vi "test_GetItemInformationFromProjects.vi"() -> (3 "Pass?":bool)   [LabVIEW 2019, in "Tests.SolutionBuilder.lvlib"]
uses:
  Tests.SolutionBuilder.lvlib
  SolutionBuilder/SolutionBuilder.lvclass
  SolutionBuilder/ProjectItem/ProjectItem.lvclass
panel:
  out "test results":u32 format="%03b"
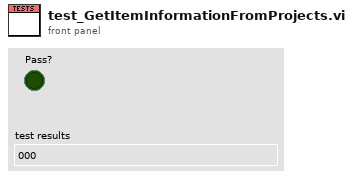
[diagram p1: front panel]
types:
  T1 = cluster{"Relative Path from 1 to 2":path, string[]}
  T2 = cluster{"Relative Path from 1 to 2":path, string[]}[]
  T3 = typedef "SolutionBuilder.lvlib/SolutionBuilder.lvclass/ProjectItemMap.ctl" = map{path, refnum<class "ProjectItem.lvclass">[]}
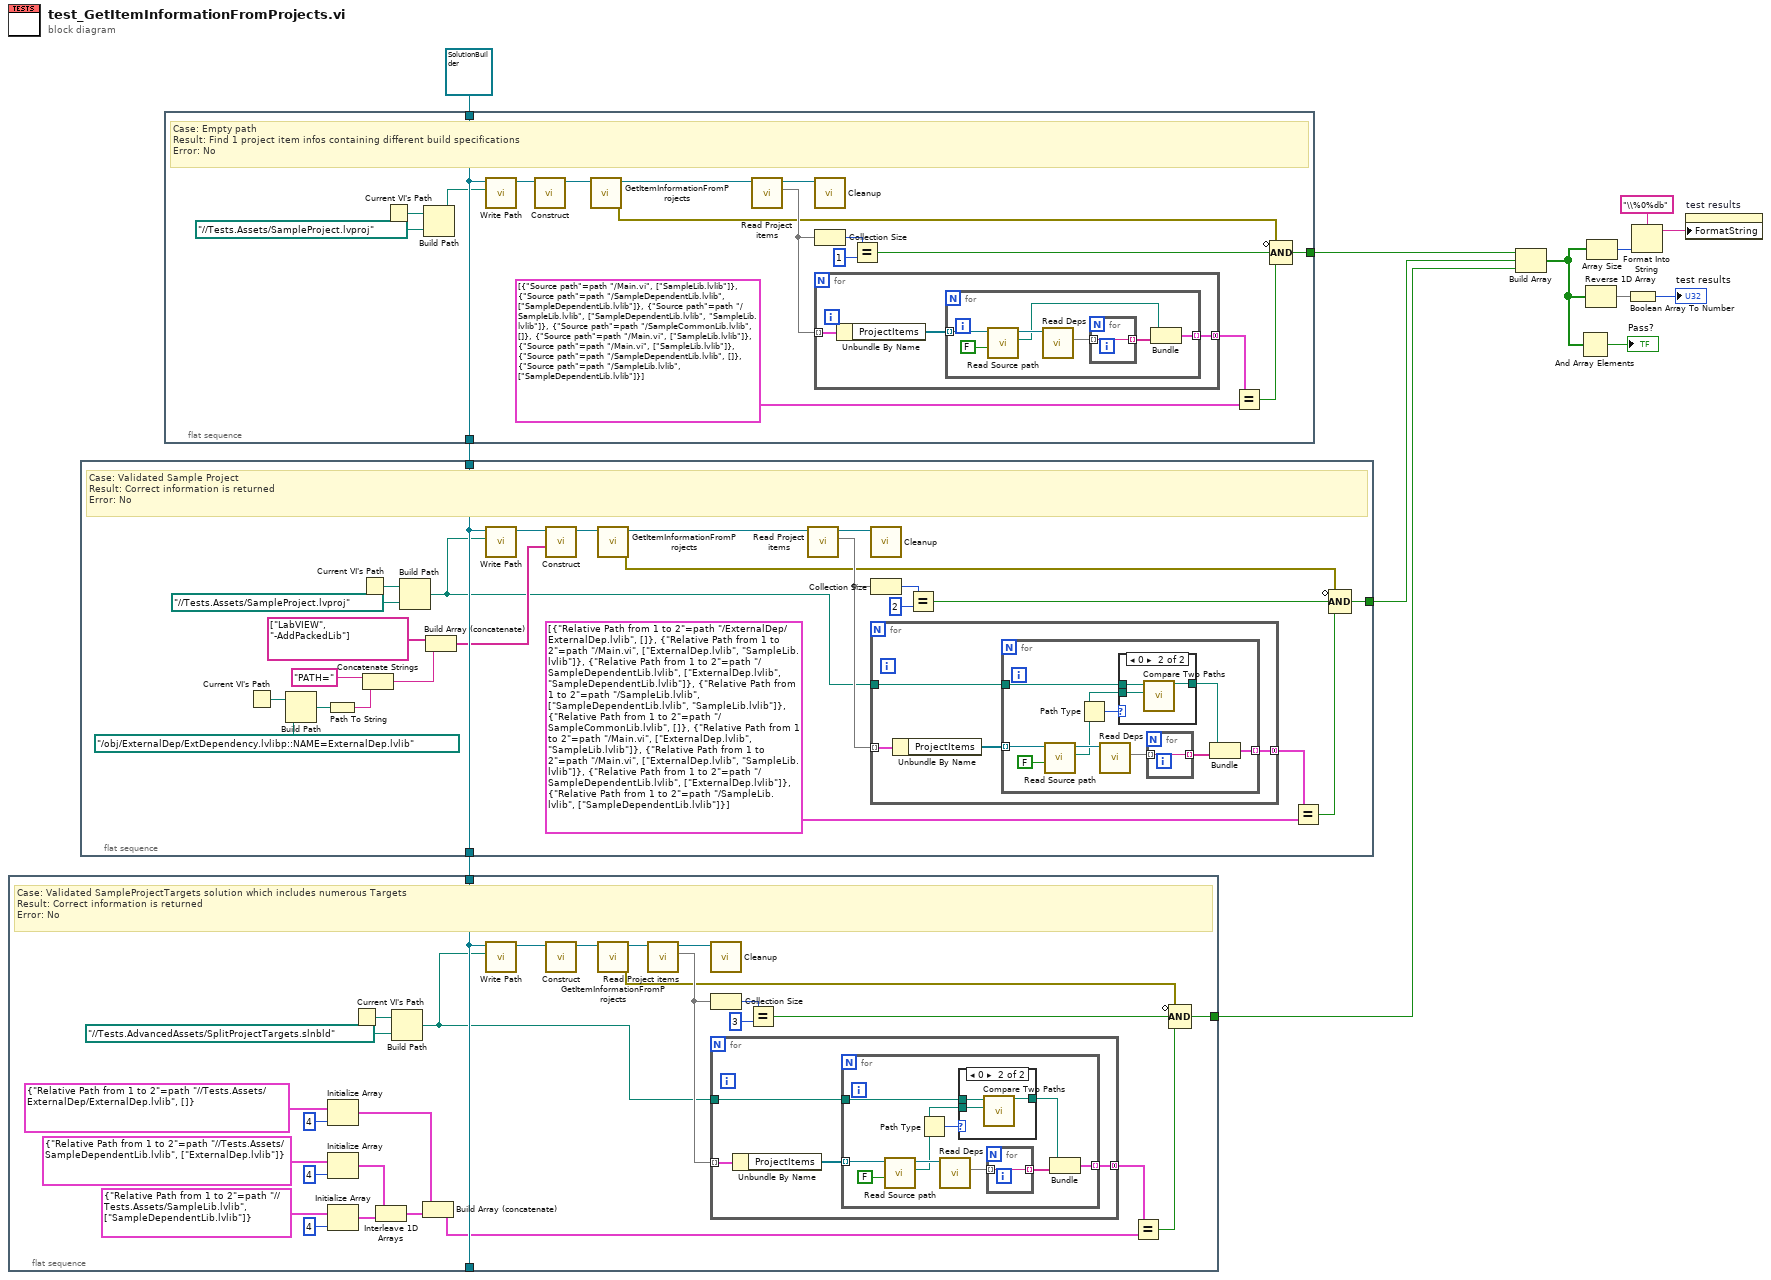
[diagram p0: block diagram]
diagram:
  n1 = flat-sequence {
    tunnel: [w33] -> w1
    tunnel: w2 -> [w40]
    tunnel: [w40] -> _
    frame #0 {
      # "Case: Validated SampleProjectTargets solution which includes numerous Targets\nResult: Correct information is returned\nError: No"
      n2 = Initialize Array(T1 {"Relative Path from 1 to 2"=path "../../Tests.Assets/ExternalDep/ExternalDep.lvlib", []}, 4 ("dimension size")) -> (w16:T2)
      n3 = Initialize Array(T1 {"Relative Path from 1 to 2"=path "../../Tests.Assets/SampleDependentLib.lvlib", ["ExternalDep.lvlib"]}, 4 ("dimension size")) -> (w18:T2)
      n4 = Initialize Array(T1 {"Relative Path from 1 to 2"=path "../../Tests.Assets/SampleLib.lvlib", ["SampleDependentLib.lvlib"]}, 4 ("dimension size")) -> (w17:T2)
      n5 = Current VI's Path() -> (path=w39:path)
      n6 = Interleave 1D Arrays(w18, w17) -> (w15:T2)
      n7 = Build Path(base path=w39, name or relative path=path "../../Tests.AdvancedAssets/SplitProjectTargets.slnbld" ("Path")) -> (appended path=w26:path)
      n8 = Build Array (concatenate)(w16, w15) -> (w14:T2)
      n9 = call-dynamic "Write Path.vi"("Path"=w26, "SolutionBuilder in"=w40) -> ("SolutionBuilder out"=w32:refnum<class "SolutionBuilder.lvclass">)  [unwired: 9 in]
      n10 = call-dynamic "Construct.vi"("SolutionBuilder in"=w32) -> ("SolutionBuilder out"=w29:refnum<class "SolutionBuilder.lvclass">)  [unwired: 9 in, 1 out]
      n11 = call-dynamic "GetItemInformationFromProjects.vi"("SolutionBuilder in"=w29) -> ("error out"=w25:errorcluster, "SolutionBuilder out"=w28:refnum<class "SolutionBuilder.lvclass">)  [unwired: 9 in]
      n12 = call-dynamic "Read Project items.vi"("SolutionBuilder in"=w28) -> ("Project items"=w35:T3, "SolutionBuilder out"=w31:refnum<class "SolutionBuilder.lvclass">)  [unwired: 9 in]
      n13 = call-dynamic "Cleanup.vi"("SolutionBuilder in"=w31) -> ()  [unwired: 9 in, 2 out]
      n14 = Collection Size(1:w35) -> (0:w37:i32)
      n15 = for {
        tunnel: w35 -> [w44] mode=indexing
        tunnel: [w42] -> w27 mode=concatenating
        tunnel: w26 -> [w41]
        n16 = Unbundle By Name(w44) -> ("ProjectItems"=w43:refnum<class "ProjectItem.lvclass">[])
        n17 = for {
          tunnel: w43 -> [w51] mode=indexing
          tunnel: [w52] -> w42 mode=indexing
          tunnel: w41 -> [w45]
          n18 = call-dynamic "Read Source path.vi"("Force abs path? (T)"=FALSE, "ProjectItem in"=w51) -> ("Source path"=w46:path, "ProjectItem out"=w50:refnum<class "ProjectItem.lvclass">)  [unwired: 8 in]
          n19 = Path Type(1:w46) -> (0:w48:i16)
          n20 = call-dynamic "Read Deps.vi"("ProjectItem in"=w50) -> ("Deps"=w54:set{string})  [unwired: 9 in, 1 out]
          n21 = case shown="0" w48 {
            tunnel: w46 -> [w55 w56]
            tunnel: [w55 w58] -> w47
            tunnel: w45 -> [_ w57]
            frame Default {
            }
            frame 0 {
              n22 = call <vilib>:"Compare Two Paths.vi"("Path 2"=w56, "Path 1"=w57) -> ("Relative Path from 1 to 2"=w58:path)  [unwired: 6 in, 3 out]
            }
          }
          n23 = for {
            tunnel: w54 -> [w59] mode=indexing
            tunnel: [w59] -> w53 mode=indexing
          }
          n24 = Bundle("Relative Path from 1 to 2"=w47, w53) -> (w52:T1)  [unwired: 1 in]
        }
      }
      n25 = Equal?(x=w37, y=3) -> (x = y?=w34:bool)
      n26 = Equal?(x=w27, y=w14) -> (x = y?=w30:bool)
      n27 = Compound Arithmetic op=AND(invert w25, w34, w30) -> (w33:bool)
    }
  }
  n28 = flat-sequence {
    tunnel: [w77] -> w3
    tunnel: w4 -> [w84]
    tunnel: [w84] -> w2
    frame #0 {
      # "Case: Validated Sample Project\nResult: Correct information is returned\nError: No"
      n29 = Current VI's Path() -> (path=w70:path)
      n30 = Build Path(base path=w70, name or relative path=path "../obj/ExternalDep/ExtDependency.lvlibp::NAME=ExternalDep.lvlib" ("Path")) -> (appended path=w72:path)
      n31 = Path To String(path=w72) -> (string=w63:string)
      n32 = Current VI's Path() -> (path=w83:path)
      n33 = Concatenate Strings("PATH=" ("string"), w63) -> (w61:string)
      n34 = Build Path(base path=w83, name or relative path=path "../../Tests.Assets/SampleProject.lvproj" ("Path")) -> (appended path=w65:path)
      n35 = Build Array (concatenate)(string[] ["LabVIEW", "-AddPackedLib"] ("App.Args"), w61) -> (w71:string[])
      n36 = call-dynamic "Write Path.vi"("Path"=w65, "SolutionBuilder in"=w84) -> ("SolutionBuilder out"=w76:refnum<class "SolutionBuilder.lvclass">)  [unwired: 9 in]
      n37 = call-dynamic "Construct.vi"("App.Args"=w71, "SolutionBuilder in"=w76) -> ("SolutionBuilder out"=w68:refnum<class "SolutionBuilder.lvclass">)  [unwired: 8 in, 1 out]
      n38 = call-dynamic "GetItemInformationFromProjects.vi"("SolutionBuilder in"=w68) -> ("error out"=w60:errorcluster, "SolutionBuilder out"=w67:refnum<class "SolutionBuilder.lvclass">)  [unwired: 9 in]
      n39 = call-dynamic "Read Project items.vi"("SolutionBuilder in"=w67) -> ("Project items"=w79:T3, "SolutionBuilder out"=w75:refnum<class "SolutionBuilder.lvclass">)  [unwired: 9 in]
      n40 = call-dynamic "Cleanup.vi"("SolutionBuilder in"=w75) -> ()  [unwired: 9 in, 2 out]
      n41 = Collection Size(1:w79) -> (0:w81:i32)
      n42 = for {
        tunnel: w79 -> [w88] mode=indexing
        tunnel: [w86] -> w66 mode=concatenating
        tunnel: w65 -> [w85]
        n43 = Unbundle By Name(w88) -> ("ProjectItems"=w87:refnum<class "ProjectItem.lvclass">[])
        n44 = for {
          tunnel: w87 -> [w95] mode=indexing
          tunnel: [w96] -> w86 mode=indexing
          tunnel: w85 -> [w89]
          n45 = call-dynamic "Read Source path.vi"("Force abs path? (T)"=FALSE, "ProjectItem in"=w95) -> ("Source path"=w90:path, "ProjectItem out"=w94:refnum<class "ProjectItem.lvclass">)  [unwired: 8 in]
          n46 = Path Type(1:w90) -> (0:w92:i16)
          n47 = call-dynamic "Read Deps.vi"("ProjectItem in"=w94) -> ("Deps"=w98:set{string})  [unwired: 9 in, 1 out]
          n48 = case shown="0" w92 {
            tunnel: w90 -> [w99 w100]
            tunnel: [w99 w102] -> w91
            tunnel: w89 -> [_ w101]
            frame Default {
            }
            frame 0 {
              n49 = call <vilib>:"Compare Two Paths.vi"("Path 2"=w100, "Path 1"=w101) -> ("Relative Path from 1 to 2"=w102:path)  [unwired: 6 in, 3 out]
            }
          }
          n50 = for {
            tunnel: w98 -> [w103] mode=indexing
            tunnel: [w103] -> w97 mode=indexing
          }
          n51 = Bundle("Relative Path from 1 to 2"=w91, w97) -> (w96:T1)  [unwired: 1 in]
        }
      }
      n52 = Equal?(x=w81, y=2) -> (x = y?=w78:bool)
      n53 = Equal?(x=w66, y=T2 [{"Relative Path from 1 to 2"=path "../ExternalDep/ExternalDep.lvlib", []}, {"Relative Path from 1 to 2"=path "../Main.vi", ["ExternalDep.lvlib", "SampleLib.lvlib"]}, {"Relative Path from 1 to 2"=path "../SampleDependentLib.lvlib", ["ExternalDep.lvlib", "SampleDependentLib.lvlib"]}, {"Relative Path from 1 to 2"=path "../SampleLib.lvlib", ["SampleDependentLib.lvlib", "SampleLib.lvlib"]}, {"Relative Path from 1 to 2"=path "../SampleCommonLib.lvlib", []}, {"Relative Path from 1 to 2"=path "../Main.vi", ["ExternalDep.lvlib", "SampleLib.lvlib"]}, {"Relative Path from 1 to 2"=path "../Main.vi", ["ExternalDep.lvlib", "SampleLib.lvlib"]}, {"Relative Path from 1 to 2"=path "../SampleDependentLib.lvlib", ["ExternalDep.lvlib"]}, {"Relative Path from 1 to 2"=path "../SampleLib.lvlib", ["SampleDependentLib.lvlib"]}] ("Array 2")) -> (x = y?=w74:bool)
      n54 = Compound Arithmetic op=AND(invert w60, w78, w74) -> (w77:bool)
    }
  }
  n55 = flat-sequence {
    tunnel: [w112] -> w7
    tunnel: refnum<class "SolutionBuilder.lvclass"> refnum ("SolutionBuilder in") -> [w120]
    tunnel: [w120] -> w4
    frame #0 {
      # "Case: Empty path\nResult: Find 1 project item infos containing different build specifications\nError: No"
      n56 = Current VI's Path() -> (path=w119:path)
      n57 = Build Path(base path=w119, name or relative path=path "../../Tests.Assets/SampleProject.lvproj" ("Path")) -> (appended path=w117:path)
      n58 = call-dynamic "Write Path.vi"("Path"=w117, "SolutionBuilder in"=w120) -> ("SolutionBuilder out"=w111:refnum<class "SolutionBuilder.lvclass">)  [unwired: 9 in]
      n59 = call-dynamic "Construct.vi"("SolutionBuilder in"=w111) -> ("SolutionBuilder out"=w107:refnum<class "SolutionBuilder.lvclass">)  [unwired: 9 in, 1 out]
      n60 = call-dynamic "GetItemInformationFromProjects.vi"("SolutionBuilder in"=w107) -> ("error out"=w104:errorcluster, "SolutionBuilder out"=w106:refnum<class "SolutionBuilder.lvclass">)  [unwired: 9 in]
      n61 = call-dynamic "Read Project items.vi"("SolutionBuilder in"=w106) -> ("Project items"=w114:T3, "SolutionBuilder out"=w109:refnum<class "SolutionBuilder.lvclass">)  [unwired: 9 in]
      n62 = call-dynamic "Cleanup.vi"("SolutionBuilder in"=w109) -> ()  [unwired: 9 in, 2 out]
      n63 = Collection Size(1:w114) -> (0:w116:i32)
      n64 = for {
        tunnel: w114 -> [w123] mode=indexing
        tunnel: [w121] -> w108 mode=concatenating
        n65 = Unbundle By Name(w123) -> ("ProjectItems"=w122:refnum<class "ProjectItem.lvclass">[])
        n66 = for {
          tunnel: w122 -> [w127] mode=indexing
          tunnel: [w128] -> w121 mode=indexing
          n67 = call-dynamic "Read Source path.vi"("Force abs path? (T)"=FALSE, "ProjectItem in"=w127) -> ("Source path"=w125:path, "ProjectItem out"=w126:refnum<class "ProjectItem.lvclass">)  [unwired: 8 in]
          n68 = call-dynamic "Read Deps.vi"("ProjectItem in"=w126) -> ("Deps"=w130:set{string})  [unwired: 9 in, 1 out]
          n69 = for {
            tunnel: w130 -> [w131] mode=indexing
            tunnel: [w131] -> w129 mode=indexing
          }
          n70 = Bundle("Source path"=w125, w129) -> (w128:cluster{"Source path":path, string[]})  [unwired: 1 in]
        }
      }
      n71 = Equal?(x=w116, y=1) -> (x = y?=w113:bool)
      n72 = Equal?(x=w108, y=cluster{"Source path":path, string[]}[] [{"Source path"=path "../Main.vi", ["SampleLib.lvlib"]}, {"Source path"=path "../SampleDependentLib.lvlib", ["SampleDependentLib.lvlib"]}, {"Source path"=path "../SampleLib.lvlib", ["SampleDependentLib.lvlib", "SampleLib.lvlib"]}, {"Source path"=path "../SampleCommonLib.lvlib", []}, {"Source path"=path "../Main.vi", ["SampleLib.lvlib"]}, {"Source path"=path "../Main.vi", ["SampleLib.lvlib"]}, {"Source path"=path "../SampleDependentLib.lvlib", []}, {"Source path"=path "../SampleLib.lvlib", ["SampleDependentLib.lvlib"]}] ("Array")) -> (x = y?=w110:bool)
      n73 = Compound Arithmetic op=AND(invert w104, w113, w110) -> (w112:bool)
    }
  }
  n74 = Build Array(w7, w3, w1) -> (w11:bool[])
  n75 = And Array Elements(Boolean array=w11) -> (logical AND=→"Pass?":bool)
  n76 = Reverse 1D Array(array=w11) -> (reversed array=w6:bool[])
  n77 = Array Size(array=w11) -> (size(s)=w9:i32)
  n78 = Boolean Array To Number(Boolean array=w6) -> (number=→"test results":u32)
  n79 = Format Into String(format string="\\%0%db", w9) -> (resulting string=w8:string)  [unwired: 2 in, 1 out]
  n80 = property on="test results" class="DigNum (strict)"("FormatString"=w8) -> ()  [unwired: 2 in, 2 out]
